vi "set_numeric.vi"(11 "output cluster 2":T1) -> (3 "output cluster":T1)   [LabVIEW 2013]
uses:
  control_ref_cluster.ctl
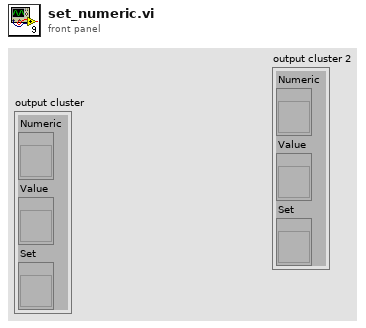
[diagram p1: front panel]
types:
  T1 = typedef "control_ref_cluster.ctl" = cluster{"Numeric":refnum<vi>, "Value":refnum<vi>, "Set":refnum<vi>}
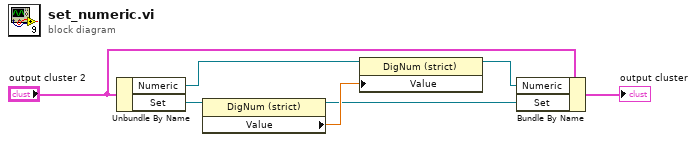
[diagram p0: block diagram]
diagram:
  n1 = Unbundle By Name("output cluster 2") -> ("Numeric"=w6:refnum<vi>, "Set"=w7:refnum<vi>)
  n2 = property class="DigNum (strict)"(reference=w7) -> (reference out=w1:refnum<vi>, "Value"=w5:dbl)  [unwired: 1 in, 1 out]
  n3 = property class="DigNum (strict)"(reference=w6, "Value"=w5) -> (reference out=w2:refnum<vi>)  [unwired: 1 in, 1 out]
  n4 = Bundle By Name(cluster="output cluster 2", "Numeric"=w2, "Set"=w1) -> (→"output cluster":T1)
